vi "second_fp.vi"(0 "Waveform chart data":T2, 3 "Stat of sensors":T4) -> ()   [LabVIEW 2016]
panel:
  in  "Tab Control":T1(tab)
  out "Waveform Chart":T2(graph)
  out "Status panel of sensors #2":T3
  in  "Remove Button":bool
  out "Vacuum,Pa":dbl(slide) scale=0.0..1.0
  out "Voltage,V":dbl(knob) scale=0.0..5.1
  out "Amperage,mA":dbl(knob) scale=0.0..35.0
  out "Pressure,kPa":dbl(slide) scale=0.0..100.0
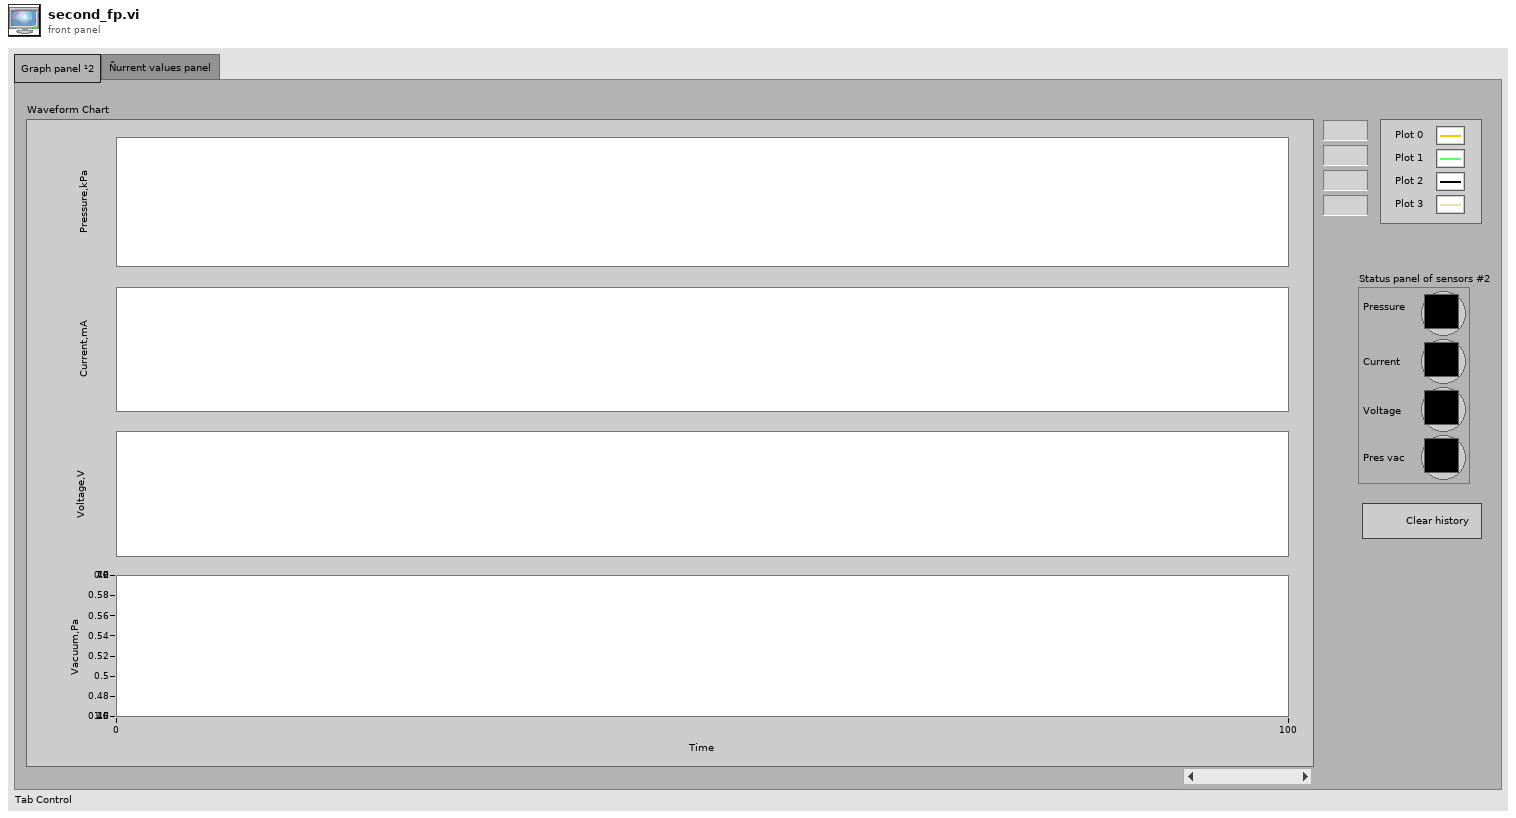
[diagram p1: front panel]
types:
  T1 = enum32{"Graph panel ¹2", "Ñurrent values panel "}
  T2 = cluster{"[0]":dbl, "[1]":dbl, "[2]":dbl, "[3]":dbl}
  T3 = cluster{"Pressure":u32, "Current":u32, "Voltage":u32, "Pres vac":u32}
  T4 = cluster{"[0]":u32, "[1]":u32, "[2]":u32, "[3]":u32}
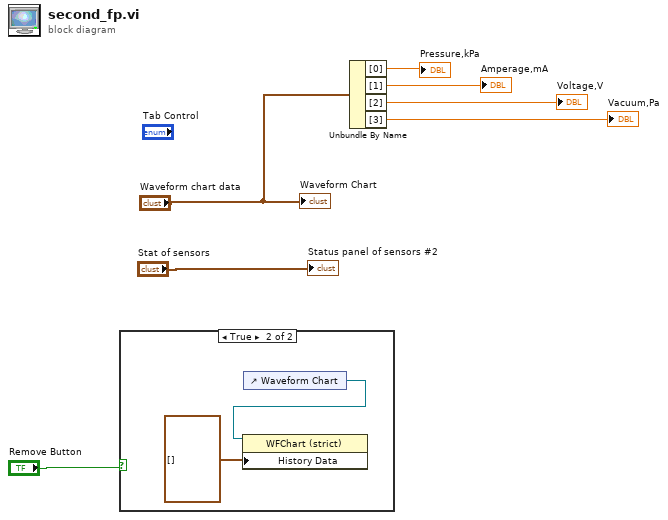
[diagram p0: block diagram]
diagram:
  n1 = case shown="True" "Remove Button" {
    frame False {
    }
    frame True {
      n2 = control-ref of="Waveform Chart"() -> (w8:refnum<vi>)
      n3 = property on="Property Node" class="WFChart (strict)"(reference=w8, "History Data"=cluster{dbl, dbl, dbl, dbl}[] []) -> ()  [unwired: 1 in, 2 out]
    }
  }
  n4 = Unbundle By Name("Waveform chart data") -> ("[0]"=→"Pressure,kPa":dbl, "[1]"=→"Amperage,mA":dbl, "[2]"=→"Voltage,V":dbl, "[3]"=→"Vacuum,Pa":dbl)
  "Waveform Chart" <- "Waveform chart data"
  "Status panel of sensors #2" <- "Stat of sensors"
